vi "Write Formats.vi"(8 "error in (no error)":errorcluster, 10 "Formats":set{T1}(c389), 11 "ZXing Options in":refnum<class "ZXing.lvclass">) -> (0 "error out":errorcluster, 3 "ZXing Options out":refnum<class "ZXing.lvclass">)   [LabVIEW 2020, in "feature_detection.lvlib" / "ZXing.lvclass"]
uses:
  ZXing.lvclass
  Format.ctl
  ZXing.lvclass/ZXing.ctl
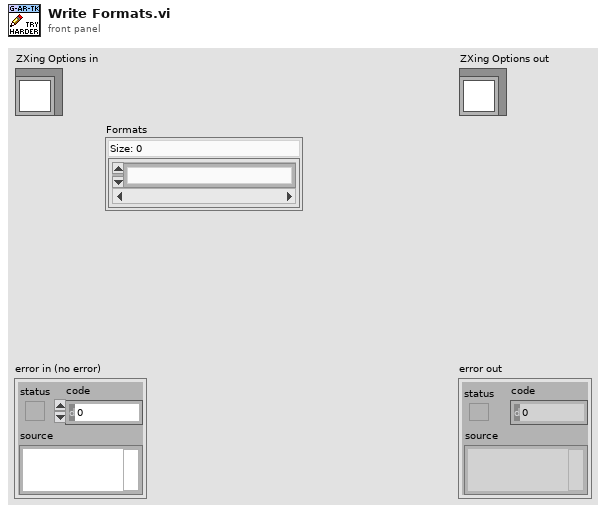
[diagram p1: front panel]
types:
  T1 = typedef "feature_detection.lvlib/ZXing.lvclass/Format.ctl" = enum8{"Aztec", "Codabar", "Code 39", "Code 93", "Code 128", "Data Bar", "Data Bar Expanded", "Data Matrix", "EAN 8", "EAN 13", "ITF", "Maxi Code", "PDF417", "QR Code", "UPCA", "UPCE", "Micro QR Code", "RM QR Code", "DX Film Edge", "Data Bar Limited"}
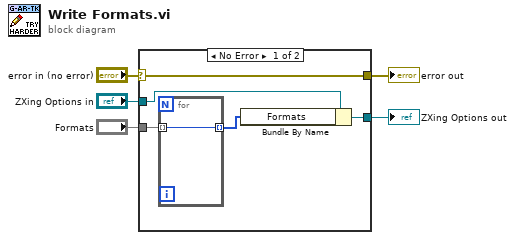
[diagram p0: block diagram]
diagram:
  n1 = case shown="No Error" "error in (no error)" {
    selector: "error in (no error)" -> [w10 w12]
    tunnel: [w10 w12] -> w4
    tunnel: [w8 w13] -> w2
    tunnel: "ZXing Options in" -> [w9 w13]
    tunnel: "Formats" -> [w6 _]
    frame No Error {
      n2 = for {
        tunnel: [w11] -> w7 mode=indexing
        tunnel: w6 -> [w11] mode=indexing
      }
      n3 = Bundle By Name(cluster=w9, "Formats"=w7) -> (w8:refnum<class "ZXing.lvclass">)
    }
    frame Error {
    }
  }
  "error out" <- w4
  "ZXing Options out" <- w2
